vi "Setup Exposure.vi"(8 "Error IN":errorcluster, 10 "Shutter":refnum<vi>, 11 "hCamera IN":u32) -> (0 "Error OUT":errorcluster, 3 "phCamera OUT":u32)   [LabVIEW 2014]
uses:
  <vilib>/addons/PixeLINK/Low Level Functions/CAMERA_FEATURES.llb/TDPU-CameraFeatures-FeatureIds.ctl
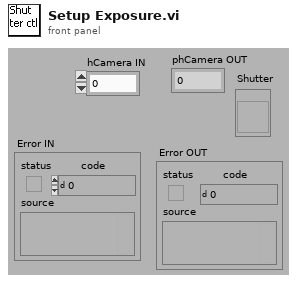
[diagram p1: front panel]
types:
  T1 = typedef "TDPU-CameraFeatures-FeatureIds.ctl" = u32
  T2 = typedef "TDPU-CameraFeatures-Camera_Feature.ctl" = cluster{"uFeatureId":T1, "uFlags":u32, "fMinValues":dbl[], "fMaxValues":dbl[]}
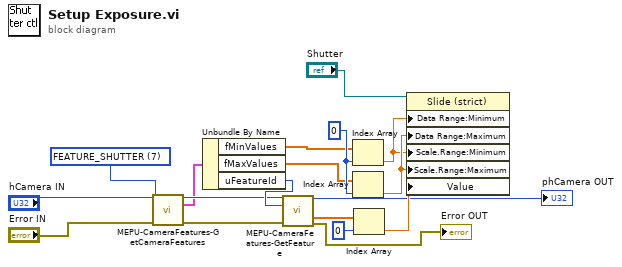
[diagram p0: block diagram]
diagram:
  w6 = T1 7 items=["FEATURE_BRIGHTNESS", "FEATURE_EXPOSURE", "FEATURE_SHARPNESS", "FEATURE_WHITE_BAL", "FEATURE_HUE", "FEATURE_SATURATION", "FEATURE_GAMMA", "FEATURE_SHUTTER", "FEATURE_GAIN", "FEATURE_IRIS", "FEATURE_FOCUS", "FEATURE_TEMPERATURE", "FEATURE_TRIGGER", "FEATURE_ZOOM", "FEATURE_PAN", "FEATURE_TILT", "FEATURE_OPT_FILTER", "FEATURE_GPIO", "FEATURE_FRAME_RATE", "FEATURE_ROI", "FEATURE_FLIP", "FEATURE_DECIMATION", "FEATURE_PIXEL_FORMAT", "FEATURE_EXTENDED_SHUTTER", "FEATURE_AUTO_ROI", "FEATURE_LOOKUP_TABLE", "FEATURE_MEMORY_CHANNEL", "FEATURE_ALL"] ("uFeatureId IN")
  w18 = 0 ("index")
  n1 = call <vilib>:"MEPU-CameraFeatures-GetCameraFeatures.vi"("hCamera IN"="hCamera IN", "uFeatureId IN"=w6, "Error IN"="Error IN") -> ("hCamera OUT"=w11:u32, "CAMERA_FEATURE"=w9:T2, "Error OUT"=w10:errorcluster)  [unwired: 10 out]
  n2 = Unbundle By Name(w9) -> ("fMinValues"=w7:dbl[], "fMaxValues"=w8:dbl[], "uFeatureId"=w12:T1)
  n3 = call <vilib>:"MEPU-CameraFeatures-GetFeature.vi"("hCamera IN"=w11, "uFeatureId IN"=w12, "Error IN"=w10) -> ("hCamera OUT"=→"phCamera OUT":u32, "pParms OUT"=w13:dbl[], "Error OUT"=→"Error OUT":errorcluster)  [unwired: 1 in, 9 out]
  n4 = Index Array(array=w7, index=w18) -> (element=w16:dbl)
  n5 = Index Array(array=w8, index=w18) -> (element=w17:dbl)
  n6 = Index Array(array=w13, index=0) -> (element=w15:dbl)
  n7 = property on="Property Node" class="Slide (strict)"(reference="Shutter", "Data Range:Minimum"=w16, "Data Range:Maximum"=w17, "Scale.Range:Minimum"=w16, "Scale.Range:Maximum"=w17, "Value"=w15) -> ()  [unwired: 1 in, 2 out]
